vi "open.vi"(8 "error in (no error)":errorcluster, 10 "flags":T1[](array[typedef]) items=["O_RDONLY", "O_WRONLY", "O_RDWR"], 11 "pathname":string) -> (0 "error out":errorcluster, 3 "file descriptor":i32)   [LabVIEW 2013, in "Linux RT IPC.lvlib" / "Pipes.lvlib"]
uses:
  Pipes.lvlib
  Controls/fcntl-linux file modes.ctl
  Controls/functions.ctl
  <vilib>/NI/NI Linux RT Errno/Linux Errno.lvlib
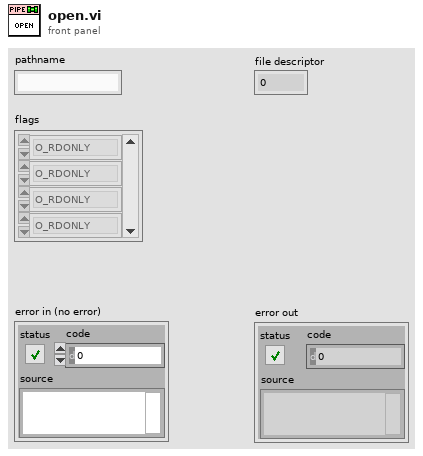
[diagram p1: front panel]
types:
  T1 = typedef "Linux RT IPC.lvlib/Pipes.lvlib/fcntl-linux file modes.ctl" = u16
  T2 = typedef "Linux RT IPC.lvlib/Pipes.lvlib/functions.ctl" = enum16{"unspecified", "mkfifo", "open", "read", "write", "close", "unlink"}
  T3 = typedef "Linux Errno.lvlib/errno.ctl" = enum16{"NO ERROR", "EPERM", "ENOENT", "ESRCH", "EINTR", "EIO", "ENXIO", "E2BIG", "ENOEXEC", "EBADF", "ECHILD", "EAGAIN", "ENOMEM", "EACCES", "EFAULT", "ENOTBLK", "EBUSY", "EEXIST", "EXDEV", "ENODEV", "ENOTDIR", "EISDIR", "EINVAL", "ENFILE", "EMFILE", "ENOTTY", "ETXTBSY", "EFBIG", "ENOSPC", "ESPIPE", "EROFS", "EMLINK", "EPIPE", "EDOM", "ERANGE", "EDADLK", "ENAMETOOLONG", "ENOLCK", "ENOSYS", "ENOTEMPTY", "ELOOP", "EWOULDBLOCK", "ENOMSG", "EIDRM", "ECHRNG", "EL2NSYNC", "EL3HLT", "EL3RST", "ELNRNG", "EUNATCH", "ENOCSI", "EL2HLT", "EBADE", "EBADR", "EXFULL", "ENOANO", "EBADRQC", "EBADSLT", "EDEADLOCK", "EBFONT", "ENOSTR", "ENODATA", "ETIME", "ENOSR", "ENONET", "ENOPKG", "EREMOTE", "ENOLINK", "EADV", "ESRMNT", "ECOMM", "EPROTO", "EMULTIHOP", "EDOTDOT", "EBADMSG", "EOVERFLOW", "ENOTUNIQ", "EBADFD", "EREMCHG", "ELIBACC", "ELIBBAD", "ELIBSCN", "ELIBMAX", "ELIBEXEC", "ELISEQ", "ERESTART", "ESTRPIPE", "EUSERS", "ENOTSOCK", "EDESTADDRREQ", "EMSGSIZE", "EPROTOTYPE", "ENOPROTOOPT", "EPROTONOSUPPORT", "ESOCKTNOSUPPORT", "EOPNOTSUPP", "EPFNOSUPPORT", "EAFNOSUPPORT", "EADDRINUSE", "EADDRNOTAVAIL", "ENETDOWN", "ENETUNREACH", "ENETRESET", "ECONNABORTED", "ECONNRESET", "ENOBUFS", "EISCONN", "ENOTCONN", "ESHUTDOWN", "ETOOMANYREFS", "ETIMEDOUT", "ECONNREFUSED", "EHOSTDOWN", "EHOSTUNREACH", "EALREADY", "EINPROGRESS", "ESTALE", "EUCLEAN", "ENOTNAM", "ENAVAIL", "EISNAM", "EREMOTEIO", "EDQUOT", "ENOMEDIUM", "EMEDIUMTYPE", "ECANCELED", "ENOKEY", "EKEYEXPIRED", "EKEYREVOKED", "EKEYREJECTED", "EOWNERDEAD", "ENOTRECOVERABLE", "ERFKILL", "EHWPOISON", "UNDEFINED"}
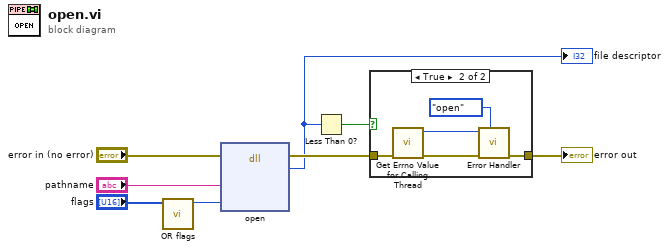
[diagram p0: block diagram]
diagram:
  n1 = call "OR flags.vi"("flags"="flags") -> ("OR'ed flags"=w5:u16)  [unwired: 10 in]
  n2 = dll-call lib="LabVIEW" fn="open"(error in="error in (no error)", "pathname"="pathname", "flags"=w5) -> (error out=w4:errorcluster, "return"=w1:i32)  [unwired: 4 in, 1 out]
  "file descriptor" <- w1
  n3 = Less Than 0?(x=w1) -> (x < 0?=w2:bool)
  n4 = case shown="True" w2 {
    tunnel: w4 -> [w9 w14]
    tunnel: [w9 w12] -> w3
    frame False {
    }
    frame True {
      n5 = call <vilib>:"Get Errno Value for Calling Thread.vi"("error in (no error)"=w14) -> ("error out"=w10:errorcluster, "errno"=w11:T3)  [unwired: 9 in]
      n6 = call "Error Handler.vi"("function (unspecified)"=functions."open", "error in (no error)"=w10, "errno"=w11) -> ("error out"=w12:errorcluster)  [unwired: 8 in]
    }
  }
  "error out" <- w3
